vi "Balancing Controller.vi"(6 "Configuration":T1={"Accelerometer Bias"={"X (m/s)"=0.0, "Y (m/s)"=0.0, "Z (m/s)"=0.0}, "Gyroscope Bias"={"X (m/s)"=0.0, "Y (m/s)"=0.0, "Z (m/s)"=0.0}, "Steering Motor Gear Ratio"=611.0, "Steering Pully Gear Ratio"=1.0, "Steering Encoder CPR"=500.0, "Steering Motor Max RPM"=4000.0, "Wheelbase (m)"=1.12, "Fork Angle (rad)"=1.3, "Balancing Controller"={"Kp (/s)"=1.0, "Kd (1)"=1.0}, "Max Allowed Steering Angle (rad)"=0.7, "Task Periods"={"Emergency Stop (us)"=10000, "IMU (us)"=10000, "Steering Motor Encoder (us)"=10000, "State Estimator (us)"=10000, "Balancing Controller (us)"=10000, "GNSS (us)"=10000, "Logging (us)"=50000, "Drive Motor (us)"=100000}, "Drive Motor Gear Ratio"=0.7, "lr"=0.4964, "lf"=0.5986, "lambda"=1.2217, "k1"=0.004472, "k2"=0.09678, "e1_max"=11.331, "Ad_t"=0.95971, "Bd_t"=0.01, "C_t"=2.20588, "D_t"=0.0, "Wheel radius"=0.311}, 8 "Measurement In":refnum<data-value>, 9 "State Estimate In":refnum<data-value>, 10 "Trajectory In":refnum<data-value>, 11 "Error In":errorcluster) -> (0 "Measurement Out":refnum<data-value>, 1 "State Estimate Out":refnum<data-value>, 3 "Error Out":errorcluster, 4 "Steering Angle Rate (rad/s)":dbl)   [LabVIEW 2021]
uses:
  State Estimator/State Estimate.ctl
  State Estimator/Measurements.ctl
  IMU/IMU Data.ctl
  Steering Motor Encoder/Steering Motor Encoder Data.ctl
  GNSS/GNSS Data.ctl
  Trajectory Control/Trajectory_Control.ctl
  Configuration/Configuration.ctl
  Logging/Log Level.ctl
panel:
  out "Trajectory Out":refnum<data-value>
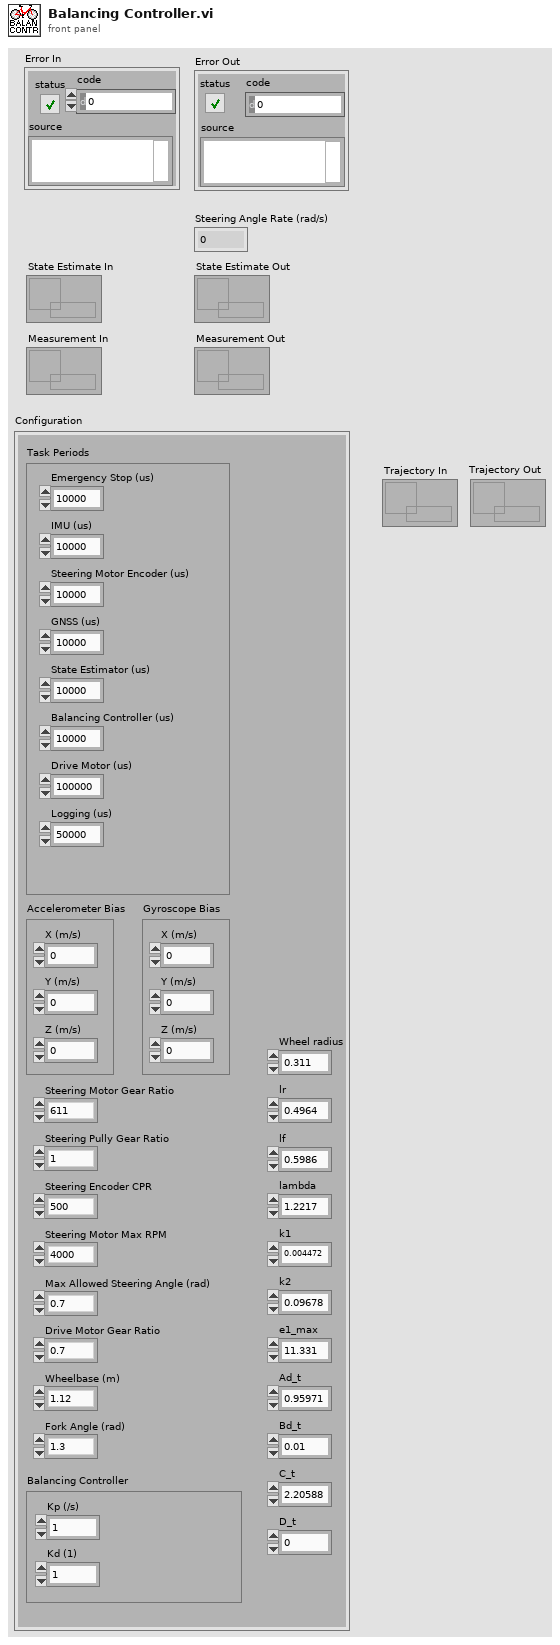
[diagram p1: front panel]
types:
  T1 = typedef "Configuration.ctl" = cluster{"Accelerometer Bias":cluster{"X (m/s)":dbl, "Y (m/s)":dbl, "Z (m/s)":dbl}, "Gyroscope Bias":cluster{"X (m/s)":dbl, "Y (m/s)":dbl, "Z (m/s)":dbl}, "Steering Motor Gear Ratio":dbl, "Steering Pully Gear Ratio":dbl, "Steering Encoder CPR":dbl, "Steering Motor Max RPM":dbl, "Wheelbase (m)":dbl, "Fork Angle (rad)":dbl, "Balancing Controller":cluster{"Kp (/s)":dbl, "Kd (1)":dbl}, "Max Allowed Steering Angle (rad)":dbl, "Task Periods":cluster{"Emergency Stop (us)":i64, "IMU (us)":i64, "Steering Motor Encoder (us)":i64, "State Estimator (us)":i64, "Balancing Controller (us)":i64, "GNSS (us)":i64, "Logging (us)":i64, "Drive Motor (us)":i64}, "Drive Motor Gear Ratio":dbl, "lr":dbl, "lf":dbl, "lambda":dbl, "k1":dbl, "k2":dbl, "e1_max":dbl, "Ad_t":dbl, "Bd_t":dbl, "C_t":dbl, "D_t":dbl, "Wheel radius":dbl}
  T2 = typedef "Log Level.ctl" = enum16{"Error", "Warning", "Info"}
  T3 = typedef "Trajectory_Control.ctl" = cluster{"Rollref":dbl, "Closestpoint":dbl, "Error1":dbl, "Error2":dbl, "Dpsiref_cont":dbl, "Lateral_cont":dbl, "Heading_cont":dbl, "Reset_traj":dbl}
  T4 = typedef "State Estimate.ctl" = cluster{"X (m)":dbl, "Y (m)":dbl, "Psi (rad)":dbl, "Roll (rad)":dbl, "Roll Rate (rad/s)":dbl, "delta":dbl, "velocity":dbl}
  T5 = typedef "Measurements.ctl" = cluster{"IMU Data":T6, "Steering Motor Encoder Data":T7, "GNSS Data":T8}
  T6 = typedef "IMU Data.ctl" = cluster{"Gyroscope":cluster{"X (rad/s)":dbl, "Y (rad/s)":dbl, "Z (rad/s)":dbl}, "Accelerometer":cluster{"X (m/s^2)":dbl, "Y (m/s^2)":dbl, "Z (m/s^2)":dbl}, "Flag IMU":dbl}
  T7 = typedef "Steering Motor Encoder Data.ctl" = cluster{"Encoder Position (counts)":i32, "Steering Angle (rad)":dbl, "Flag Steering Encoder":dbl}
  T8 = typedef "GNSS Data.ctl" = cluster{"Latitude (rad)":dbl, "Longitude (rad)":dbl, "Altitude (m)":dbl, "Speed (m/s)":dbl, "Heading (rad)":dbl, "Fix Quality":i32, "Number of Satellites":i32, "Latitude (deg)":dbl, "Longitude (deg)":dbl, "Flag GNSS":dbl}
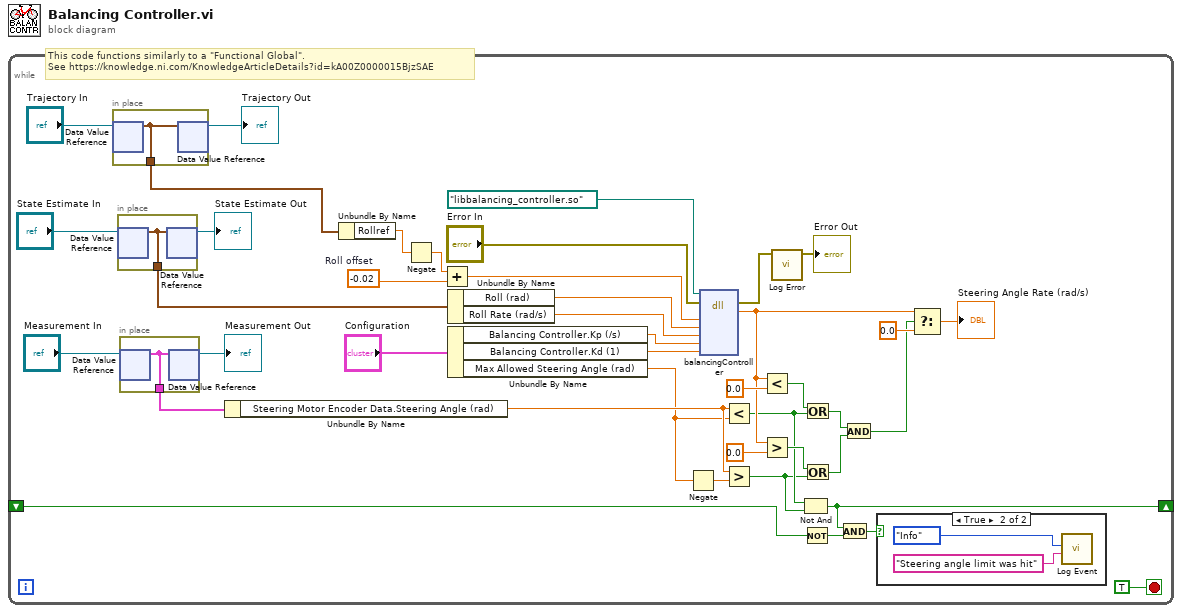
[diagram p0: block diagram]
diagram:
  # "This code functions similarly to a \"Functional Global\".\nSee https://knowledge.ni.com/KnowledgeArticleDetails?id=kA00Z0000015BjzSAE"
  n1 = while {
    shift-right: [w11] -> _
    shift-left: _ -> [w13]
    stop <- TRUE stop-if-true
    w5 = -0.02  # Roll offset
    n2 = in-place {
      in-place-border: [w43] -> w4
      n3 = in-place-dvr #1 ("Data Value Reference Read / Write Element")("Trajectory In") -> (w43:T3)  [unwired: 1 out]
      n4 = in-place-dvr #1(w43) -> (→"Trajectory Out":refnum<data-value>)  [unwired: 1 out]
    }
    n5 = in-place {
      in-place-border: [w47] -> w34
      n6 = in-place-dvr #2("State Estimate In") -> (w47:T4)  [unwired: 1 out]
      n7 = in-place-dvr #2(w47) -> (→"State Estimate Out":refnum<data-value>)  [unwired: 1 out]
    }
    n8 = in-place {
      in-place-border: [w46] -> w31
      n9 = in-place-dvr #3("Measurement In") -> (w46:T5)  [unwired: 1 out]
      n10 = in-place-dvr #3(w46) -> (→"Measurement Out":refnum<data-value>)  [unwired: 1 out]
    }
    n11 = Unbundle By Name(w31) -> ("Steering Motor Encoder Data.Steering Angle (rad)"=w19:dbl)
    n12 = Unbundle By Name(w4) -> ("Rollref"=w2:dbl)
    n13 = Negate(x=w2) -> (-x=w1:dbl)
    n14 = Add(x=w1, y=w5) -> (x+y=w6:dbl)
    n15 = Unbundle By Name(w34) -> ("Roll (rad)"=w39:dbl, "Roll Rate (rad/s)"=w38:dbl)
    n16 = Unbundle By Name("Configuration") -> ("Balancing Controller.Kp (/s)"=w37:dbl, "Balancing Controller.Kd (1)"=w36:dbl, "Max Allowed Steering Angle (rad)"=w18:dbl)
    n17 = Negate(x=w18) -> (-x=w20:dbl)
    n18 = dll-call lib="?" fn="balancingController"(path in=path "libbalancing_controller.so", error in="Error In", "rollReference"=w6, "roll"=w39, "rollRate"=w38, "Kp"=w37, "Kd"=w36) -> (error out=w16:errorcluster, "Steering Angle Rate"=w24:dbl)  [unwired: 6 in, 1 out]
    n19 = Less?(x=w19, y=w18) -> (x < y?=w10:bool)
    n20 = Greater?(x=w19, y=w20) -> (0:w9:bool)
    n21 = Less?(x=w24, y=0.0) -> (x < y?=w27:bool)
    n22 = Greater?(x=w24, y=0.0) -> (0:w23:bool)
    n23 = call "Log Error.vi"("Error In"=w16) -> ("Error Out"=→"Error Out":errorcluster)  [unwired: 10 in]
    n24 = Not And(1:w9, 2:w10) -> (0:w11:bool)
    n25 = Not(x=w13) -> (.not. x?=w14:bool)
    n26 = Or(x=w27, y=w10) -> (x .or. y?=w26:bool)
    n27 = Or(x=w23, y=w9) -> (x .or. y?=w22:bool)
    n28 = And(x=w11, y=w14) -> (x .and. y?=w12:bool)
    n29 = And(x=w26, y=w22) -> (x .and. y?=w21:bool)
    n30 = case shown="True" w12 {
      frame False {
      }
      frame True {
        n31 = call "Log Event.vi"("Message"="Steering angle limit was hit", "Log Level"=Log_Level."Info") -> ()  [unwired: 9 in, 1 out]
      }
    }
    n32 = Select(t=w24, s=w21, f=0.0) -> (s? t:f=→"Steering Angle Rate (rad/s)":dbl)
  }
